vi "Grabber Control.vi"(8 "Arm Motor Exhale Tote":bool, 9 "Arm Motor Inhale Tote":bool) -> ()   [LabVIEW 2014]
panel:
  out "error out":errorcluster
  out "Motor Output Grabber":dbl
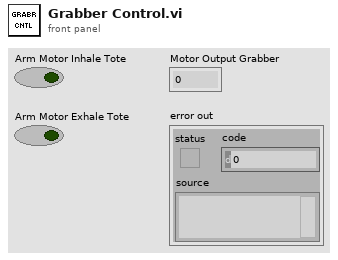
[diagram p1: front panel]
types:
  T1 = typedef "WPI_MotorControlDeviceRef.ctl" = cluster{"DeviceStatus":errorcluster, "Type":T2, "PWM":cluster{"Controller":T3, "PWM Channel":T4, "DeadBand":T5}, "CAN":cluster{"Device Number":u8, "Control Mode":T6, "Semaphore":T7, "Max Vout":dbl, "TalonSRX Control Mode":T8}, "Invert":bool, "TransformRef":T9, "InvTransformRef":T9}
  T2 = typedef "WPI_MotorControlType.ctl" = enum16{"PWM", "CAN", "CANTalonSRX"}
  T3 = typedef "FPGA_TypedefDigitalModule.ctl" = enum16{"Controller 1"}
  T4 = typedef "FPGA_DIOPWMChannel.ctl" = enum8{"PWM 0", "PWM 1", "PWM 2", "PWM 3", "PWM 4", "PWM 5", "PWM 6", "PWM 7", "PWM 8", "PWM 9", "PWM MXP 0", "PWM MXP 1", "PWM MXP 2", "PWM MXP 3", "PWM MXP 4", "PWM MXP 5", "PWM MXP 6", "PWM MXP 7", "PWM MXP 8", "PWM MXP 9", "Invalid"}
  T5 = typedef "WPI_PWMDeadband.ctl" = cluster{"Name":string, "maxPositivePwm":i32, "minPositivePwm":i32, "centerPwm":i32, "maxNegativePwm":i32, "minNegativePwm":i32, "angularRange":u16}
  T6 = typedef "WPI_CANJaguar_ControlMode.ctl" = enum8{"Percent VBus", "Current", "Speed", "Position", "Voltage"}
  T7 = typedef "Semaphore RefNum" = refnum<k1>
  T8 = typedef "WPI_CANTalonSRX_APIControlMode.ctl" = enum8{"Percent VBus", "Speed", "Position", "Slave", "Unchanged / Invalid"}
  T9 = typedef "WPI_PWMTransform_ConPane.ctl" = refnum<vi>
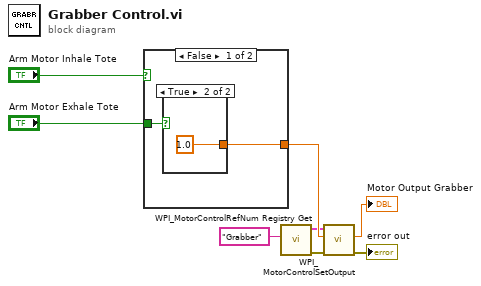
[diagram p0: block diagram]
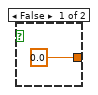
[diagram p2: hidden frame]
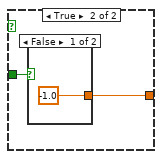
[diagram p3: hidden frame]
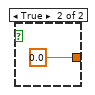
[diagram p4: hidden frame]
diagram:
  n1 = case shown="False" "Arm Motor Inhale Tote" {
    tunnel: "Arm Motor Exhale Tote" -> [w10 w14]
    tunnel: [w9 w13] -> w5
    frame False {
      n2 = case shown="True" w10 {
        tunnel: [0.0 ("Output") 1.0 ("Output")] -> w9
        frame False {
        }
        frame True {
        }
      }
    }
    frame True {
      n3 = case shown="False" w14 {
        tunnel: [-1.0 ("Output") 0.0 ("Output")] -> w13
        frame False {
        }
        frame True {
        }
      }
    }
  }
  n4 = call <vilib>:"WPI_MotorControlRefNum Registry Get.vi"("refnum name"="Grabber") -> ("error out"=w7:errorcluster, "MotorControlDevRef"=w4:T1)  [unwired: 9 in]
  n5 = call <vilib>:"WPI_MotorControlSetOutput.vi"("error in (no error)"=w7, "Output"=w5, "MotorControlDevRef"=w4) -> ("error out"=→"error out":errorcluster, "Motor Output"=→"Motor Output Grabber":dbl)  [unwired: 6 in, 1 out]
